vi "Saccade suppression - moving grating by time.vi"() -> ()   [LabVIEW 2013]
uses:
  <vilib>/Platform/TimedLoop/XDataNode/timing_clust.ctl
  <vilib>/Platform/TimedLoop/XDataNode/nitl_modes.ctl
  <vilib>/Platform/TimedLoop/XDataNode/wakeup.ctl
  <vilib>/gmath/statdist.llb/Uniform (Discrete) Random.vi
  Eye tracking dependencies/Global 1.vi
  <vilib>/platform/TimedLoop/XDataNode/XDataNode.xnode
  <vilib>/Platform/TimedLoop/XDataNode/XDNodeRunTimeDep.lvlib
  <vilib>/gmath/NI_Gmath.lvlib
panel:
  out "Eye tracker":bool
  out "Std name":string="70915_animal15-21_exp1"
  out "Blank":bool
  out "Total number of trials":i32=2
  out "Running!":bool=TRUE
  in  "Location":string="E:\\Beh_Data\\"
  out "File name exists!":bool
  out "Current trial #":u16=1
  out "LED":bool
  in  "Abort":bool caption="run-stop"
  in  "File name":string="17"
  in  "Save data":bool
  out "State Missed":bool
  out "VS missed":bool
  out "State busy":bool=TRUE
  out "VS busy":bool=TRUE
  in  "Tab Control":T1(tab)=enum."Network"
  in  "Notes":string
  in  "Start recording @":string
  in  "Inserted probe @":string
  in  "Brain region":string
  in  "Anesthesia @":string
  in  "Anesthesia":string
  in  "Probe configuration":string
  in  "Probe use number":string
  in  "Probe ID":string
  in  "Probe type":string
  in  "Electrode spacing":string
  in  "Electrode area":string
  in  "Penetration angle (to pia)":string
  in  "Penetration coordinates":string
  in  "Penetration distance":string
  in  "Penetration number":string
  in  "Genotype":string
  in  "Transfection":string
  in  "Mass":string
  in  "Sex":string
  in  "Age":string
  in  "Animal ID":string="14-4"
  in  "inter flash interval (ms)":dbl=500.0
  in  "Max jitter (ms)":dbl=500.0
  in  "VS type":string="saccade_grating"
  in  "Background luminance":sgl=40.0
  in  "Pulse amp 0":sgl
  in  "Pulse amp 1":sgl
  in  "Pulse delay (ms)":sgl
  in  "Pulse width (ms)":sgl
  in  "Pulse period":sgl
  in  "Pulse #":sgl
  in  "LED mode":u16(ring) items=["No LED", "Random"]
  in  "Chance (%)":dbl
  in  "# of trials":i32=1
  in  "run-stop":bool=TRUE
  in  "Time (min)":sgl=1.0
  in  "Flash luminance":sgl=100.0
  in  "flash duration (ms)":dbl=16.0
  in  "VS subtype":string="movingByTime"
  in  "Include blanks":bool=TRUE
  in  "# of blank trials":i32=1
  in  "7":bool
  in  "6":bool
  in  "5":bool
  in  "4":bool
  in  "3":bool
  in  "2":bool
  in  "1":bool
  in  "0":bool=TRUE
  in  "Temporal Frequency":sgl=2.0
  in  "Contrast":sgl=1.0
  in  "Spatial Frequency":sgl=0.03
  in  "Give reward":bool
  in  "Manually give shock":bool
  in  "Water duration (ms)":u32=30
  in  "Shock duration (ms)":u32=10
  in  "Water refractory period (ms)":u32=500
  in  "Shock refractory period (ms)":u32=1000
  in  "Trial timeout (ms)":u32=3000
  in  "Track eye":bool=TRUE
  in  "Allow shock":bool
  in  "Allow timeout":bool
  in  "Manually give water":bool
  in  "Reward period (ms)":u32
  in  "Reward start delay (ms)":u32
  in  "Lick threshold (V)":fxp<+,32,16>=1.600006103515625
  in  "VS threshold (V)":fxp<+,32,16>=0.5
  out "Originating IP":string="192.168.137.2"
  out "Incoming data":string="TrlDone 1.000 "
  in  "Update cycle (ms)":dbl=50.0
  in  "Local IP_This computer":string="192.168.137.10"
  in  "Remote IP_Broadcast":string="192.168.137.255"
  in  "Remote IP_State machine":string="192.168.137.2"
  in  "Remote IP_Visual stimulation":string="192.168.137.3"
  in  "Local port":u16=9090
  in  "Remote port":u16=9091
  out "Error 2":string
  # "Saccade suppression project"
  # "Current trial"
  # "of"
  # "System Status"
  # "VS"
  # "State machine"
  # "Busy"
  # "Missed trial"
  # "Max 20 characters"
  # "(w/o LED)"
  # "Time per trial (min)"
  # "MAX 199.9988"
  # "(% of blank trials that have LED)"
  # "Errors for debugging"
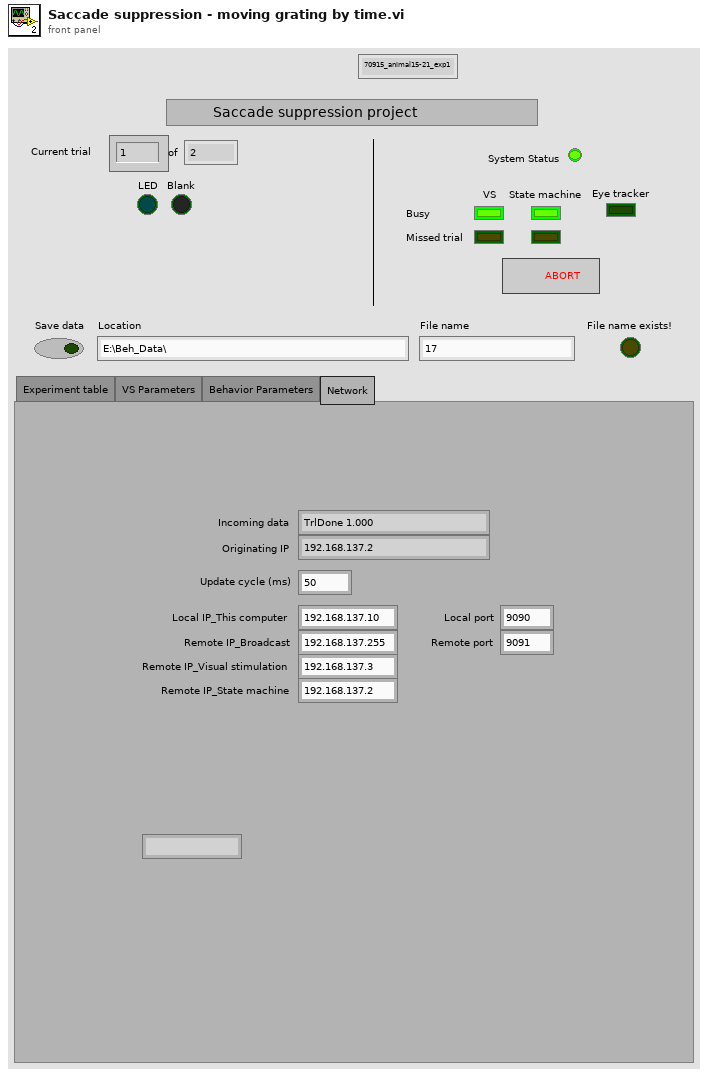
[diagram p1: front panel]
types:
  T1 = enum32{"Experiment table", "VS Parameters", "Behavior Parameters", "Network"}
  T2 = typedef "XDNodeRunTimeDep.lvlib/timing_clust.ctl" = cluster{"Expected End [f-1]":u64, "Actual End [f-1]":u64, "Finished Late? [f-1]":bool, "Expected End [i-1]":u64, "Actual End [i-1]":u64, "Finished Late? [i-1]":bool, "Expected Start [i]":u64, "Actual Start [i]":u64, "Expected Start [f]":u64, "Actual Start [f]":u64, "Source Name":string, "Structure Name":string, "Period":i64, "Deadline":i64, "Offset":i64, "Start":i64, "Priority":i32, "Timeout":i32, "Mode":T3, "Wakeup Reason":T4, "Error":errorcluster, "Source Type":string, "Secondary Source Type":string, "Global End Time":u64, "Global Start Time":u64, "Frame Duration":u64, "Iteration Duration":u64, "Assigned CPU":i32, "I/O Scan Engine Mode":u32}
  T3 = typedef "XDNodeRunTimeDep.lvlib/nitl_modes.ctl" = enum32{"No Change", "Process missed periods, maintain original phase", "Discard missed periods, maintain original phase", "Process missed periods, ignore original phase", "Discard missed periods, ignore original phase"}
  T4 = typedef "XDNodeRunTimeDep.lvlib/wakeup.ctl" = enum32{"Normal", "Aborted", "Asynchronous wakeup", "Timing source error", "Timed loop error", "Timeout"}
  T5 = enum16{"big-endian, network order", "native, host order", "little-endian"}
  T6 = enum16{"open", "replace", "create", "open or create", "replace or create", "replace or create with confirmation"}
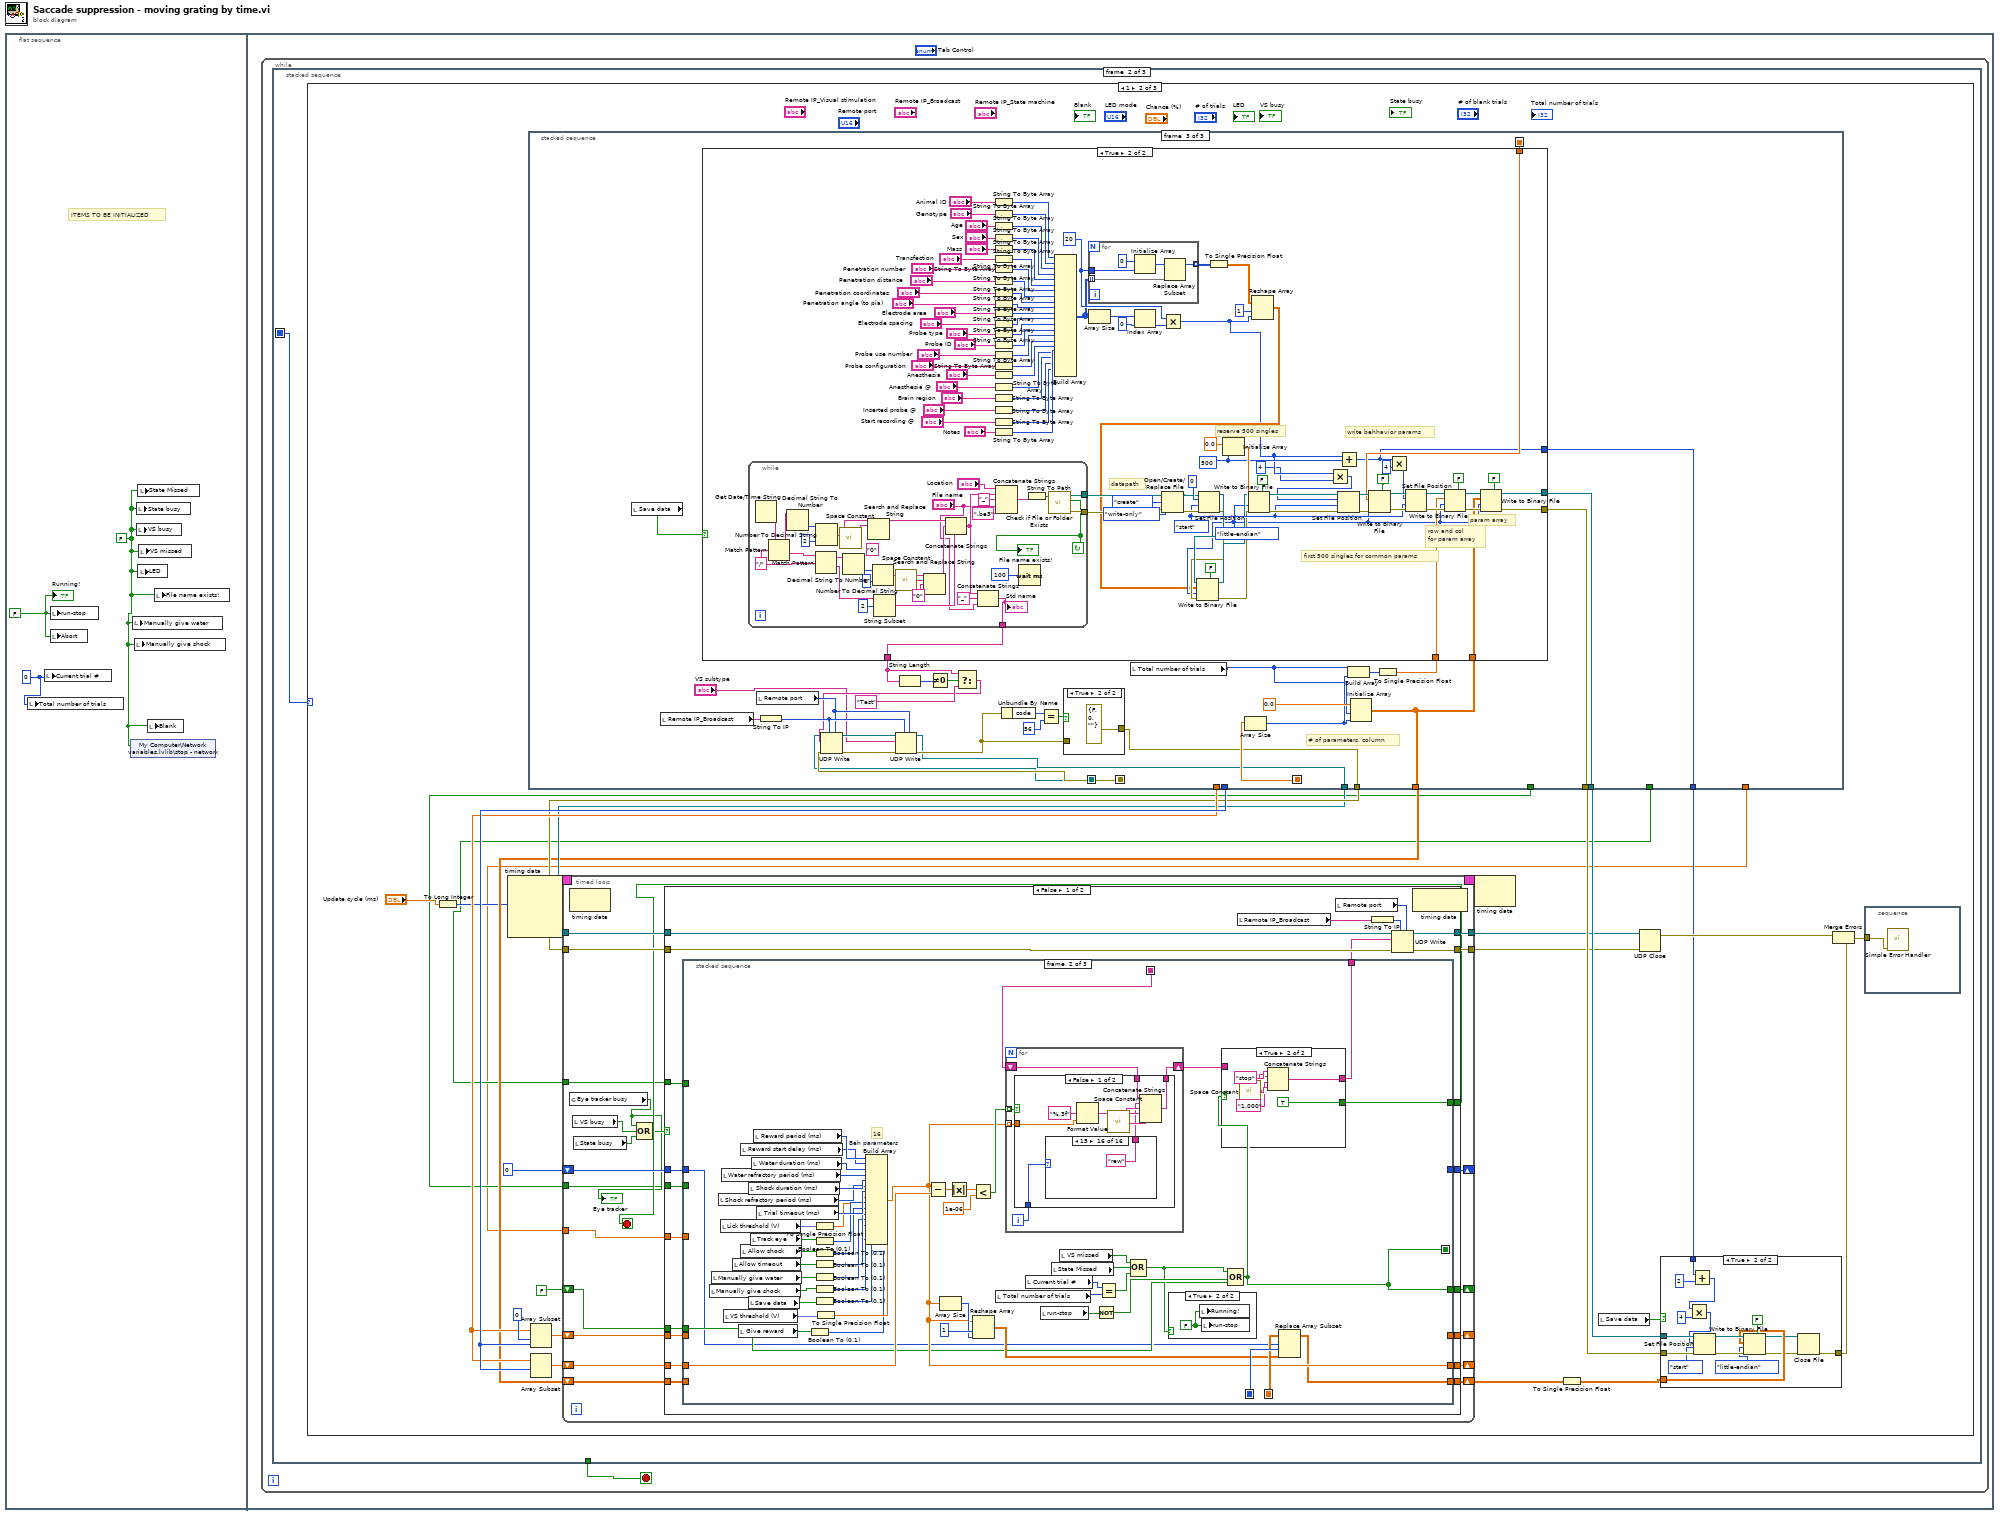
[diagram p0: block diagram]
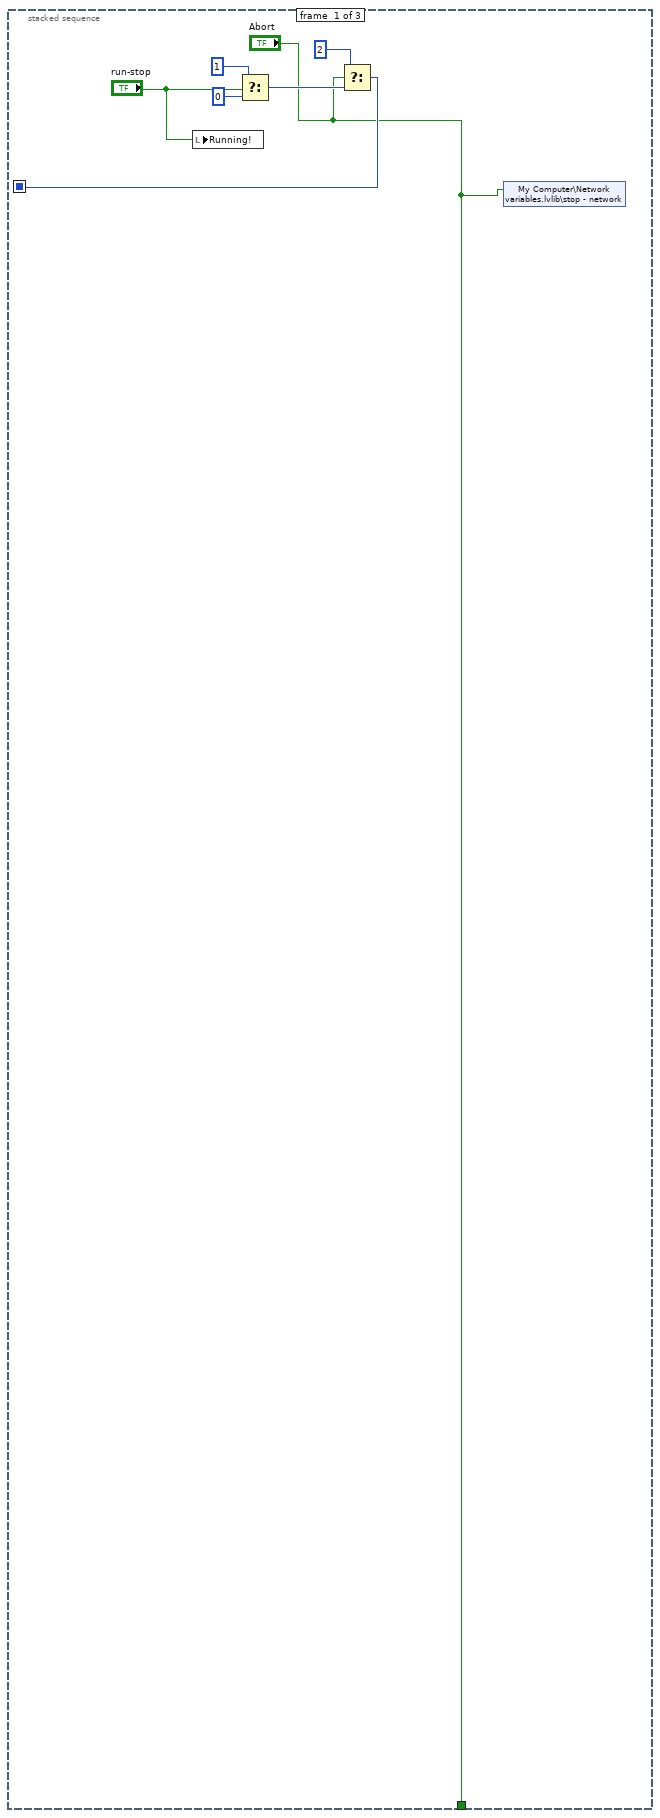
[diagram p2: hidden frame]
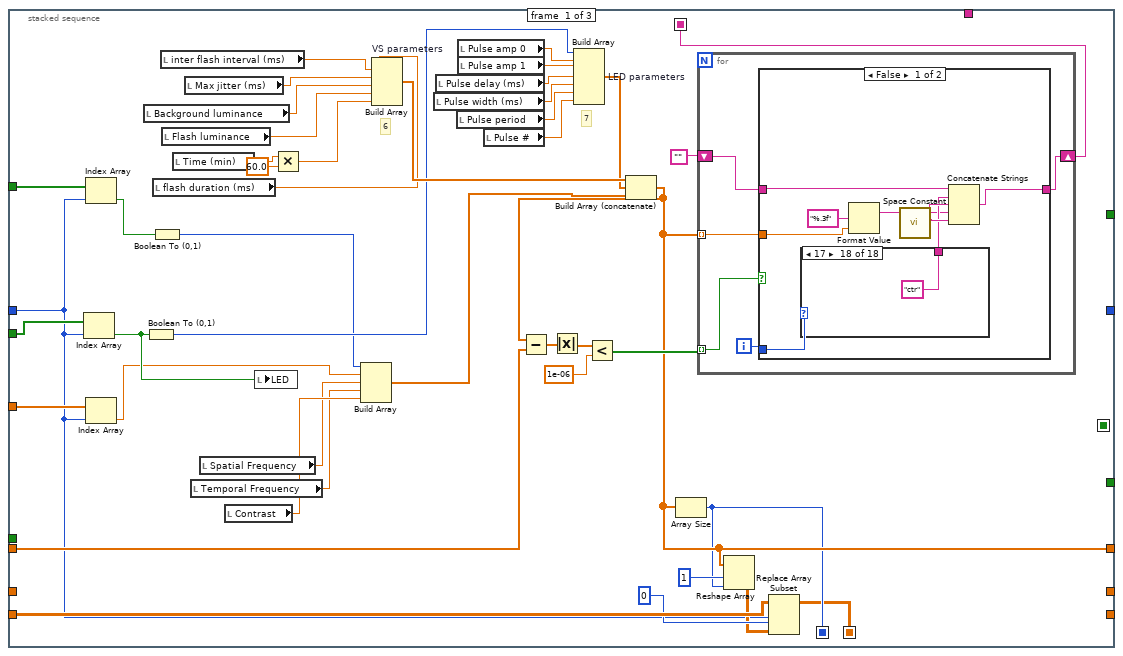
[diagram p4: hidden frame]
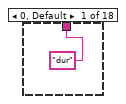
[diagram p5: hidden frame]
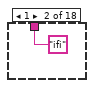
[diagram p6: hidden frame]
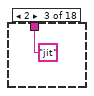
[diagram p7: hidden frame]
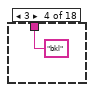
[diagram p8: hidden frame]
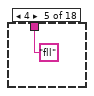
[diagram p9: hidden frame]
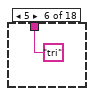
[diagram p10: hidden frame]
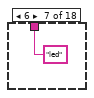
[diagram p11: hidden frame]
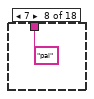
[diagram p12: hidden frame]
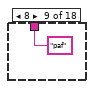
[diagram p13: hidden frame]
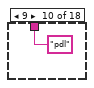
[diagram p14: hidden frame]
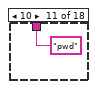
[diagram p15: hidden frame]
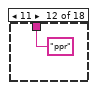
[diagram p16: hidden frame]
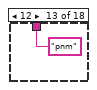
[diagram p17: hidden frame]
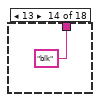
[diagram p18: hidden frame]
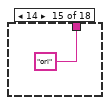
[diagram p19: hidden frame]
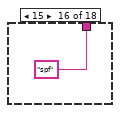
[diagram p20: hidden frame]
diagram:
  n1 = flat-sequence {
    frame #0 {
      w2 = u16 0
      w1 = FALSE ("L dist ind")
      w3 = FALSE
      # "ITEMS TO BE INITIALIZED"
      n2 = local write "Total number of trials"(w2) -> ()
      n3 = local write "Current trial #"(w2) -> ()
      n4 = local write "run-stop"(w3) -> ()
      n5 = local write "Abort"(w3) -> ()
      n6 = shared-variable "My Computer\\Network variables.lvlib\\stop - network"(w1) -> ()  [unwired: 1 in, 1 out]
      n7 = local write "Manually give water"(w1) -> ()
      n8 = local write "Manually give shock"(w1) -> ()
      n9 = local write "State busy"(w1) -> ()
      n10 = local write "VS busy"(w1) -> ()
      n11 = local write "State Missed"(w1) -> ()
      n12 = local write "LED"(w1) -> ()
      n13 = local write "VS missed"(w1) -> ()
      n14 = local write "Blank"(w1) -> ()
      n15 = local write "File name exists!"(w1) -> ()
      "Running!" <- w3
    }
    frame #1 {
      n16 = while {
        stop <- w4 stop-if-true
        n17 = stacked-sequence {
          seq-local: [w7 _ _] -> [_ w12 _]
          tunnel: ["Abort" _ _] -> w4
          frame #0 {
            n18 = local write "Running!"("run-stop") -> ()
            n19 = Select(t=u8 1, s="run-stop", f=u8 0) -> (s? t:f=w8:u8)
            n20 = Select(t=u8 2, s="Abort", f=w8) -> (s? t:f=w7:u8)
            n21 = shared-variable "My Computer\\Network variables.lvlib\\stop - network"("Abort") -> ()  [unwired: 1 in, 1 out]
          }
          frame #1 {
            n22 = case shown="1" w12 {
              frame 0, Default {
              }
              frame 1 {
                n23 = To Long Integer(number="Update cycle (ms)") -> (32bit integer=w23:i32)
                n24 = node-c288(w23) -> (w40:T2)  [unwired: 3 in]
                n25 = stacked-sequence {
                  seq-local: [w464 _ _] -> [_ _ w676]
                  seq-local: [_ w618 _] -> [_ _ w667]
                  seq-local: [w473 _ _] -> [_ _ w665]
                  seq-local: [w472 _ _] -> [_ _ w651]
                  tunnel: [w464 _ _] -> w35
                  tunnel: [w461 _ _] -> w36
                  tunnel: [_ _ w649] -> w32
                  tunnel: [_ _ w648] -> w31
                  tunnel: [_ _ w670] -> w30
                  tunnel: [_ _ w669] -> w26
                  tunnel: [_ _ w668] -> w25
                  tunnel: [_ _ w646] -> w16
                  tunnel: [w457 _ _] -> w15
                  tunnel: [w456 _ _] -> w14
                  tunnel: [w448 _ _] -> w13
                  frame #0 {
                    # "5"
                    # "Orientation"
                    n26 = Boolean To (0,1)(Boolean="Give reward") -> (0, 1=w474:i16)
                    n27 = Boolean To (0,1)(Boolean="Track eye") -> (0, 1=w514:i16)
                    n28 = To Single Precision Float(number="Lick threshold (V)") -> (single precision float=w479:sgl)
                    n29 = Boolean To (0,1)(Boolean="Allow shock") -> (0, 1=w512:i16)
                    n30 = Boolean To (0,1)(Boolean="Allow timeout") -> (0, 1=w510:i16)
                    n31 = Boolean To (0,1)(Boolean="Manually give water") -> (0, 1=w508:i16)
                    n32 = Boolean To (0,1)(Boolean="Save data") -> (0, 1=w505:i16)
                    n33 = To Single Precision Float(number="VS threshold (V)") -> (single precision float=w476:sgl)
                    n34 = Boolean To (0,1)(Boolean="Manually give shock") -> (0, 1=w507:i16)
                    n35 = Build Array "Beh parameters 16"("Reward period (ms)", "Reward start delay (ms)", "Water duration (ms)", "Water refractory period (ms)", "Shock duration (ms)", "Shock refractory period (ms)", "Trial timeout (ms)", w479, w514, w512, w510, w508, w507, w505, w476, w474) -> (w463:sgl[])
                    n36 = local read "Remote IP_Broadcast"() -> (w492:string)
                    n37 = String To IP(1:"Local IP_This computer") -> (0:w496:u32)
                    n38 = UDP Open(7:w496, 11:"Local port") -> (port=w493:refnum<k16>, 0:w497:errorcluster)  [unwired: 3 in, 1 out]
                    n39 = local read "Remote port"() -> (w487:u16)
                    n40 = Multiply(x="Time (min)", y=sgl 60.0) -> (x*y=w454:sgl)
                    n41 = String To IP(1:w492) -> (0:w488:u32)
                    n42 = Build Array "VS parameters 6"("flash duration (ms)", "inter flash interval (ms)", "Max jitter (ms)", "Background luminance", "Flash luminance", w454) -> (w483:dbl[])
                    n43 = Array Size(array=w483) -> (size(s)=w481:i32)
                    n44 = call <vilib>:"Space Constant.vi"() -> ("String"=w490:string)
                    n45 = stacked-sequence {
                      tunnel: [w525 _] -> w457
                      tunnel: [w524 _] -> w456
                      tunnel: [_ w578] -> w448
                      frame #0 {
                        n46 = case shown="True" "Include blanks" {
                          tunnel: [w529 w532] -> w525
                          tunnel: [w527 w534] -> _
                          tunnel: [w526 w533] -> w524
                          frame False {
                            n47 = local read "# of trials"() -> (w527:i32)
                            n48 = Initialize Array(FALSE, w527) -> (w526:bool[])
                            n49 = Initialize Array(FALSE, w527) -> (w529:bool[])
                            n50 = local write "Total number of trials"(w527) -> ()
                          }
                          frame True {
                            n51 = local read "LED mode"() -> (w535:u16)
                            n52 = local read "# of blank trials"() -> (w531:i32)
                            n53 = local read "# of trials"() -> (w536:i32)
                            n54 = Add(x=w536, y=w531) -> (x+y=w534:i32)
                            n55 = local write "Total number of trials"(w534) -> ()
                            n56 = Initialize Array(FALSE, w536) -> (w537:bool[])
                            n57 = for {
                              N: w531 -> [_]
                              shift-right: [w571] -> w532
                              shift-left: w537 -> [w572]
                              n58 = Array Size(array=w572) -> (size(s)=w576:i32)
                              n59 = call-poly <vilib>:"Discrete Random.vi"("n"=w576, "samples"=1) -> ("uniform (discrete) random data"=w575:i32[])  [unwired: 8 in, 1 out]
                              n60 = Index Array(array=w575, index=0) -> (element=w573:i32)
                              n61 = Decrement(x=w573) -> (x-1=w570:i32)
                              n62 = Insert Into Array(array=w572, index=w570, new element=TRUE) -> (w571:bool[])
                            }
                            n63 = case shown="1" w535 {
                              tunnel: w534 -> [w541 w543]
                              tunnel: [w540 w544] -> w533
                              tunnel: w532 -> [_ w549]
                              tunnel: w531 -> [_ _]
                              frame 0, Default {
                                n64 = Initialize Array(FALSE, w541) -> (w540:bool[])
                              }
                              frame 1 {
                                n65 = local read "Chance (%)"() -> (w547:dbl)
                                n66 = Decrement(x=w543) -> (x-1=w542:i32)
                                n67 = Divide(x=w547, y=100.0) -> (x/y=w545:dbl)
                                n68 = while {
                                tunnel: w549 -> [w557]
                                shift-right: [w555] -> w544
                                shift-left: bool[] [] -> [w554]
                                tunnel: w545 -> [w553]
                                tunnel: w542 -> [w551]
                                i -> [w552]
                                stop <- w550 stop-if-true
                                n69 = Index Array(array=w557, index=w552) -> (element=w556:bool)
                                n70 = Equal?(x=w552, y=w551) -> (x = y?=w550:bool)
                                n71 = case shown="True" w556 {
                                tunnel: [w559 w568] -> w555
                                tunnel: w554 -> [w558 w567]
                                tunnel: w553 -> [_ w562]
                                frame False {
                                n72 = Build Array (concatenate)(w558, FALSE) -> (w559:bool[])
                                }
                                frame True {
                                n73 = Random Number (0-1)() -> (number: 0 to 1=w561:dbl)
                                n74 = Less?(x=w561, y=w562) -> (x < y?=w563:bool)
                                n75 = Select(t=TRUE, s=w563, f=FALSE) -> (s? t:f=w566:bool)
                                n76 = Build Array (concatenate)(w567, w566) -> (w568:bool[])
                                }
                                }
                                }
                              }
                            }
                          }
                        }
                      }
                      frame #1 {
                        n77 = local read "Total number of trials"() -> (w580:i32)
                        n78 = for {
                          N: w580 -> [_]
                          shift-right: [w581] -> w578
                          shift-left: sgl[] [] ("array type (2D Dbl)") -> [w582]
                          n79 = Boolean To (0,1)(Boolean="6") -> (0, 1=w590:i16)
                          n80 = Boolean To (0,1)(Boolean="7") -> (0, 1=w589:i16)
                          n81 = Boolean To (0,1)(Boolean="5") -> (0, 1=w591:i16)
                          n82 = Boolean To (0,1)(Boolean="4") -> (0, 1=w592:i16)
                          n83 = Boolean To (0,1)(Boolean="0") -> (0, 1=w596:i16)
                          n84 = Boolean To (0,1)(Boolean="1") -> (0, 1=w595:i16)
                          n85 = Boolean To (0,1)(Boolean="3") -> (0, 1=w593:i16)
                          n86 = Boolean To (0,1)(Boolean="2") -> (0, 1=w594:i16)
                          n87 = Compound Arithmetic op=ADD(w596, w595, w594, w593, w592, w591, w590, w589) -> (w588:i16)
                          n88 = Build Array(w596, w595, w594, w593, w592, w591, w590, w589) -> (w587:i16[])
                          n89 = call-poly <vilib>:"Discrete Random.vi"("n"=w588, "samples"=1) -> ("uniform (discrete) random data"=w607:i32[])  [unwired: 8 in, 1 out]
                          n90 = Index Array(array=w607, index=0) -> (element=w605:i32)
                          n91 = Decrement(x=w605) -> (x-1=w586:i32)
                          n92 = while {
                            tunnel: w587 -> [w616]
                            tunnel: [w614] -> w584
                            tunnel: w586 -> [w612]
                            shift-right: [w609] -> _
                            shift-left: 0 -> [w610]
                            i -> [w613]
                            stop <- w611 stop-if-true
                            n93 = Search 1D Array(1D array=w616, element=i16 1, start index (0)=w610) -> (index of element=w614:i32)
                            n94 = Equal?(x=w613, y=w612) -> (x = y?=w611:bool)
                            n95 = Increment(x=w614) -> (x+1=w609:i32)
                          }
                          n96 = To Single Precision Float(number=w584) -> (single precision float=w583:sgl)
                          n97 = Build Array (concatenate)(w582, w583) -> (w581:sgl[])
                        }
                      }
                    }
                    n98 = Index Array(array=w448, index=0) -> (element=w450:sgl)
                    n99 = Index Array(array=w456, index=0) -> (element=w459:bool)
                    n100 = Index Array(array=w457, index=0) -> (element=w465:bool)
                    n101 = Boolean To (0,1)(Boolean=w459) -> (0, 1=w458:i16)
                    n102 = Build Array "LED parameters 7"(w458, "Pulse amp 0", "Pulse amp 1", "Pulse delay (ms)", "Pulse width (ms)", "Pulse period", "Pulse #") -> (w482:sgl[])
                    n103 = Array Size(array=w482) -> (size(s)=w480:i32)
                    n104 = Add(x=w481, y=w480) -> (x+y=w462:i32)
                    n105 = Increment(x=w462) -> (x+1=w461:i32)
                    n106 = Boolean To (0,1)(Boolean=w465) -> (0, 1=w451:i16)
                    n107 = Build Array(w451, w450, "Spatial Frequency", "Temporal Frequency", "Contrast") -> (w452:sgl[])
                    n108 = Build Array (concatenate)(w483, w482, w452, w463) -> (w464:dbl[])
                    n109 = Array To Spreadsheet String(delimiter (Tab)=w490, array=w464, 3:"%.3f" ("format string")) -> (spreadsheet string=w489:string)
                    n110 = UDP Write(address=w488, port or service name=w487, connection ID=w493, data in=w489, 8:w497) -> (error out=w486:errorcluster, 3:w485:refnum<k16>)  [unwired: 1 in]
                    n111 = UDP Write(address=w488, port or service name=w487, connection ID=w485, data in="VS type", 8:w486) -> (error out=w473:errorcluster, 3:w472:refnum<k16>)  [unwired: 1 in]
                  }
                  frame #1 {
                    w625 = "&" ("string")
                    # "state definition"
                    n112 = local read "inter flash interval (ms)"() -> (w640:dbl)
                    n113 = local read "Total number of trials"() -> (w617:i32)
                    n114 = local read "Max jitter (ms)"() -> (w639:dbl)
                    n115 = local read "VS subtype"() -> (w644:string)
                    n116 = local read "Chance (%)"() -> (w638:dbl)
                    n117 = local read "LED mode"() -> (w641:u16)
                    n118 = local read "VS type"() -> (w645:string)
                    n119 = String To Byte Array(string=w645) -> (unsigned byte array=w643:u8[])
                    n120 = String To Byte Array(string=w644) -> (unsigned byte array=w642:u8[])
                    n121 = Concatenate Strings("idle", w625, "vs before", w625, "vs", w625, "vs after", w625, "cycle end", w625, "reward", w625, "reward refractory", w625, "punish", w625, "punish refractory", w625, "exit", w625, "timeout", w625) -> (w626:string)
                    n122 = Build Array (concatenate)(w643, w642, w641, w617, w640, w639, w638) -> (w622:dbl[])
                    n123 = String To Byte Array(string=w626) -> (unsigned byte array=w620:u8[])
                    n124 = Initialize Array(sgl 0.0 ("element"), 37 ("dimension size")) -> (w621:sgl[])
                    n125 = Build Array (concatenate)(w622, w621, w620) -> (w619:dbl[])
                    n126 = To Single Precision Float(number=w619) -> (single precision float=w618:sgl[])
                  }
                  frame #2 {
                    # "# of parameters, column"
                    n127 = local read "Save data"() -> (w673:bool)
                    n128 = local read "Remote IP_Broadcast"() -> (w659:string)
                    n129 = local read "Remote port"() -> (w657:u16)
                    n130 = String To IP(1:w659) -> (0:w658:u32)
                    n131 = local read "Total number of trials"() -> (w666:i32)
                    n132 = Array Size(array=w676) -> (size(s)=w674:i32)
                    n133 = Build Array(w666, w674) -> (w672:i32[])
                    n134 = Initialize Array(sgl 0.0, w666, w674) -> (w670:sgl[][])
                    n135 = To Single Precision Float(number=w672) -> (single precision float=w671:sgl[])
                    n136 = case shown="True" w673 {
                      tunnel: w671 -> [_ w749]
                      tunnel: w670 -> [_ w748]
                      tunnel: [_ w747] -> w669
                      tunnel: [_ w746] -> w668
                      tunnel: w667 -> [_ w745]
                      tunnel: ["" w681] -> w653
                      tunnel: [_ w680] -> w646
                      frame False {
                      }
                      frame True {
                        w716 = 20 ("dimension size")
                        w686 = 500 ("dimension size")
                        w688 = T5."little-endian" ("byte order (0:big-endian, network order)")
                        w758 = enum16{"start", "end", "current"}."start" ("from (0:start)")
                        # "param array"
                        # "row and col\nfor param array"
                        # "first 500 singles for common params"
                        # "reserve 500 singles"
                        # "write behhavior params"
                        # "datapath"
                        n137 = while {
                          tunnel: [w789] -> w751
                          tunnel: [w788] -> w750
                          tunnel: [w781] -> w681
                          stop <- w786 continue-if-true
                          (unwired) "0" ("replace string (\"\")")
                          w810 = "/"
                          n138 = Get Date/Time String() -> (date string=w812:string)  [unwired: 3 in, 1 out]
                          n139 = Match Pattern(string=w812, regular expression=w810) -> (before substring=w809:string, after substring=w811:string)  [unwired: 1 in, 2 out]
                          n140 = Decimal String To Number(string=w809) -> (number=w804:i32)  [unwired: 2 in, 1 out]
                          n141 = Match Pattern(string=w811, regular expression=w810) -> (before substring=w808:string, after substring=w798:string)  [unwired: 1 in, 2 out]
                          n142 = Number To Decimal String(number=w804, width (-)=i16 2) -> (decimal integer string=w806:string)
                          n143 = call <vilib>:"Space Constant.vi"() -> ("String"=w805:string)
                          n144 = Decimal String To Number(string=w808) -> (number=w801:i32)  [unwired: 2 in, 1 out]
                          n145 = Search and Replace String(input string=w806, search string=w805) -> (result string=w796:string)  [unwired: 6 in, 3 out]
                          n146 = Number To Decimal String(number=w801, width (-)=i16 2) -> (decimal integer string=w803:string)
                          n147 = String Subset(string=w798, offset (0)=2) -> (substring=w794:string)  [unwired: 1 in]
                          n148 = call <vilib>:"Space Constant.vi"() -> ("String"=w802:string)
                          n149 = Search and Replace String(input string=w803, search string=w802, replace string="0" ("replace string (\"\")")) -> (result string=w795:string)  [unwired: 5 in, 3 out]
                          n150 = Concatenate Strings(w796, w795, w794) -> (w784:string)
                          n151 = Concatenate Strings(w784, "_" ("string"), "File name") -> (w781:string)
                          "Std name" <- w781
                          n152 = Concatenate Strings("Location", w784, "_" ("string"), "File name", ".be3" ("string")) -> (w791:string)
                          n153 = Wait (ms)(milliseconds to wait=u32 100) -> ()  [unwired: 1 out]
                          n154 = String To Path(string=w791) -> (path=w790:path)
                          n155 = call <vilib>:"Check if File or Folder Exists.vi"("path"=w790) -> ("error out"=w788:errorcluster, "file or folder exists?"=w786:bool, "dup path"=w789:path)  [unwired: 8 in]
                          "File name exists!" <- w786
                        }
                        n156 = String To Byte Array(string="Animal ID") -> (unsigned byte array=w708:u8[])
                        n157 = String To Byte Array(string="Genotype") -> (unsigned byte array=w699:u8[])
                        n158 = String To Byte Array(string="Age") -> (unsigned byte array=w700:u8[])
                        n159 = String To Byte Array(string="Sex") -> (unsigned byte array=w701:u8[])
                        n160 = String To Byte Array(string="Mass") -> (unsigned byte array=w702:u8[])
                        n161 = String To Byte Array(string="Transfection") -> (unsigned byte array=w703:u8[])
                        n162 = String To Byte Array(string="Penetration number") -> (unsigned byte array=w705:u8[])
                        n163 = String To Byte Array(string="Penetration distance") -> (unsigned byte array=w707:u8[])
                        n164 = String To Byte Array(string="Penetration coordinates") -> (unsigned byte array=w731:u8[])
                        n165 = String To Byte Array(string="Penetration angle (to pia)") -> (unsigned byte array=w732:u8[])
                        n166 = String To Byte Array(string="Electrode area") -> (unsigned byte array=w733:u8[])
                        n167 = String To Byte Array(string="Electrode spacing") -> (unsigned byte array=w734:u8[])
                        n168 = String To Byte Array(string="Probe type") -> (unsigned byte array=w735:u8[])
                        n169 = String To Byte Array(string="Probe ID") -> (unsigned byte array=w736:u8[])
                        n170 = String To Byte Array(string="Probe use number") -> (unsigned byte array=w737:u8[])
                        n171 = String To Byte Array(string="Probe configuration") -> (unsigned byte array=w738:u8[])
                        n172 = String To Byte Array(string="Anesthesia") -> (unsigned byte array=w739:u8[])
                        n173 = String To Byte Array(string="Anesthesia @") -> (unsigned byte array=w740:u8[])
                        n174 = String To Byte Array(string="Brain region") -> (unsigned byte array=w741:u8[])
                        n175 = String To Byte Array(string="Inserted probe @") -> (unsigned byte array=w742:u8[])
                        n176 = String To Byte Array(string="Start recording @") -> (unsigned byte array=w743:u8[])
                        n177 = String To Byte Array(string="Notes") -> (unsigned byte array=w744:u8[])
                        n178 = Build Array(w708, w699, w700, w701, w702, w703, w705, w707, w731, w732, w733, w734, w735, w736, w737, w738, w739, w740, w741, w742, w743, w744) -> (w711:u8[][])
                        n179 = for {
                          tunnel: w711 -> [w778] mode=indexing
                          tunnel: [w777] -> w709 mode=indexing
                          tunnel: w716 -> [w776]
                          n180 = Initialize Array(u8 0 ("element"), w776) -> (w780:u8[])
                          n181 = Replace Array Subset(array=w780, new element=w778) -> (w777:u8[])  [unwired: 1 in]
                        }
                        n182 = Array Size(array=w711) -> (size(s)=w713:i32[])
                        n183 = Index Array(array=w713, index=0) -> (element=w715:i32)
                        n184 = Open/Create/Replace File(file path (use dialog)=w751, error in=w750, operation (0:open)=T6."create", access (0:read/write)=enum16{"read/write", "read-only", "write-only"}."write-only") -> (refnum out=w772:refnum<file>, error out=w771:errorcluster)  [unwired: 2 in, 1 out]
                        n185 = Multiply(x=w716, y=w715) -> (x*y=w684:i32)
                        n186 = Set File Position(offset (in bytes) (0)=i64 0, refnum=w772, from (0:start)=w758, error in=w771) -> (refnum out=w692:refnum<file>, error out=w690:errorcluster)
                        n187 = To Single Precision Float(number=w709) -> (single precision float=w710:sgl[][])
                        n188 = Initialize Array(sgl 0.0 ("element"), w686) -> (w768:sgl[])
                        n189 = Reshape Array(w710, 1 ("dimension size"), w684) -> (w687:sgl[][])
                        n190 = Write to Binary File(file (use dialog)=w692, data=w687, error in=w690, 5:FALSE ("prepend array or string size? (T)"), 9:w688) -> (refnum out=w691:refnum<file>, error out=w689:errorcluster)  [unwired: 1 in, 1 out]
                        n191 = Write to Binary File(file (use dialog)=w691, data=w768, error in=w689, 5:FALSE ("prepend array or string size? (T)"), 9:w688) -> (refnum out=w766:refnum<file>, error out=w765:errorcluster)  [unwired: 1 in, 1 out]
                        n192 = Multiply(x=w684, y=4) -> (x*y=w685:i32)
                        n193 = Set File Position(offset (in bytes) (0)=w685, refnum=w766, from (0:start)=w758, error in=w765) -> (refnum out=w764:refnum<file>, error out=w763:errorcluster)
                        n194 = Add(x=w684, y=w686) -> (x+y=w680:i32)
                        n195 = Write to Binary File(file (use dialog)=w764, data=w745, error in=w763, 5:FALSE ("prepend array or string size? (T)"), 9:w688) -> (refnum out=w762:refnum<file>, error out=w761:errorcluster)  [unwired: 1 in, 1 out]
                        n196 = Multiply(x=w680, y=4) -> (x*y=w760:i32)
                        n197 = Set File Position(offset (in bytes) (0)=w760, refnum=w762, from (0:start)=w758, error in=w761) -> (refnum out=w756:refnum<file>, error out=w755:errorcluster)
                        n198 = Write to Binary File(file (use dialog)=w756, data=w749, error in=w755, 5:FALSE ("prepend array or string size? (T)"), 9:w688) -> (refnum out=w754:refnum<file>, error out=w753:errorcluster)  [unwired: 1 in, 1 out]
                        n199 = Write to Binary File(file (use dialog)=w754, data=w748, error in=w753, 5:FALSE ("prepend array or string size? (T)"), 9:w688) -> (refnum out=w746:refnum<file>, error out=w747:errorcluster)  [unwired: 1 in, 1 out]
                      }
                    }
                    n200 = String Length(string=w653) -> (length=w656:i32)
                    n201 = Not Equal To 0?(x=w656) -> (x != 0?=w655:bool)
                    n202 = Select(t=w653, s=w655, f="Test") -> (s? t:f=w652:string)
                    n203 = UDP Write(address=w658, port or service name=w657, connection ID=w651, data in=w652, 8:w665) -> (error out=w664:errorcluster, 3:w650:refnum<k16>)  [unwired: 1 in]
                    n204 = UDP Write(address=w658, port or service name=w657, connection ID=w650, data in="VS subtype", 8:w664) -> (error out=w660:errorcluster, 3:w648:refnum<k16>)  [unwired: 1 in]
                    n205 = Unbundle By Name(w660) -> ("code"=w663:i32)
                    n206 = Equal?(x=w663, y=56) -> (x = y?=w661:bool)
                    n207 = case shown="True" w661 {
                      tunnel: w660 -> [w677 _]
                      tunnel: [w677 errorcluster {"status"=FALSE, "code"=0, "source"=""} ("error out")] -> w649
                      frame False {
                      }
                      frame True {
                      }
                    }
                  }
                }
                n208 = Array Subset(array=w35, index=0, length=w36) -> (w38:dbl[])
                n209 = Array Subset(array=w35, index=w36) -> (w34:dbl[])  [unwired: 1 in]
                n210 = timed-loop {
                  shift-right: [w61] -> _
                  shift-left: u16 0 -> [w60]
                  tunnel: w32 -> [w59]
                  tunnel: w31 -> [w58]
                  tunnel: [w57] -> w17
                  tunnel: [w56] -> w18
                  shift-right: [w55] -> _
                  shift-left: w38 -> [w63]
                  shift-right: [w54] -> _
                  shift-left: w34 -> [w62]
                  shift-right: [w52] -> w29
                  shift-left: w30 -> [w53]
                  shift-right: [w51] -> _
                  shift-left: FALSE -> [w50]
                  timing: w40 -> [_]
                  timing-out: [_] -> w39
                  tunnel: w15 -> [w44]
                  tunnel: w14 -> [w43]
                  tunnel: w13 -> [w42]
                  stop <- w49 stop-if-true
                  n211 = node-c288() -> ()  [unwired: 1 in, 1 out]
                  n212 = global read "Global 1.vi" "Eye tracker busy"() -> (w45:bool)
                  "Eye tracker" <- w45
                  n213 = local read "VS busy"() -> (w47:bool)
                  n214 = local read "State busy"() -> (w46:bool)
                  n215 = Compound Arithmetic op=OR(w45, w47, w46) -> (w48:bool)
                  n216 = case shown="False" w48 {
                    tunnel: w63 -> [w87 w277]
                    tunnel: w62 -> [w86 w275]
                    tunnel: [w85 w266] -> w61
                    tunnel: w60 -> [w84 w267]
                    tunnel: w59 -> [w80 w273]
                    tunnel: w58 -> [w79 w271]
                    tunnel: [w78 w272] -> w57
                    tunnel: [w77 w270] -> w56
                    tunnel: [w76 w277] -> w55
                    tunnel: [w75 w268] -> w54
                    tunnel: w53 -> [w74 w276]
                    tunnel: [w73 w276] -> w52
                    tunnel: [w72 w269] -> w51
                    tunnel: w50 -> [w71 w274]
                    tunnel: [w69 FALSE] -> w49
                    tunnel: w44 -> [w68 _]
                    tunnel: w43 -> [w67 _]
                    tunnel: w42 -> [w66 _]
                    frame False {
                      n217 = stacked-sequence {
                        seq-local: [w117 _ _] -> [_ w188 _]
                        seq-local: [w110 _ _] -> [_ w182 _]
                        seq-local: [w109 _ _] -> [_ w181 _]
                        seq-local: [_ w171 _] -> [_ _ w258]
                        tunnel: w84 -> [w94 w169 w260]
                        tunnel: w87 -> [w122 _ _]
                        tunnel: w86 -> [_ w195 _]
                        tunnel: [_ _ w259] -> w85
                        tunnel: [w114 _ _] -> w76
                        tunnel: [_ w178 _] -> w75
                        tunnel: w74 -> [w113 _ _]
                        tunnel: [_ w176 _] -> w73
                        tunnel: [_ w171 _] -> w72
                        tunnel: w71 -> [_ w172 _]
                        tunnel: [_ w170 _] -> w70
                        tunnel: [_ w163 _] -> w69
                        tunnel: w68 -> [w103 _ _]
                        tunnel: w67 -> [w101 _ _]
                        tunnel: w66 -> [w95 _ _]
                        frame #0 {
                          # "6"
                          # "7"
                          n218 = Index Array(array=w101, index=w94) -> (element=w99:bool)
                          n219 = Index Array(array=w103, index=w94) -> (element=w102:bool)
                          n220 = Index Array(array=w95, index=w94) -> (element=w90:sgl)
                          n221 = local read "Background luminance"() -> (w106:sgl)
                          n222 = Boolean To (0,1)(Boolean=w99) -> (0, 1=w100:i16)
                          n223 = Boolean To (0,1)(Boolean=w102) -> (0, 1=w89:i16)
                          n224 = local read "flash duration (ms)"() -> (w104:dbl)
                          n225 = local read "inter flash interval (ms)"() -> (w108:dbl)
                          n226 = local read "Flash luminance"() -> (w105:sgl)
                          n227 = local read "Time (min)"() -> (w97:sgl)
                          n228 = local read "Max jitter (ms)"() -> (w107:dbl)
                          n229 = local read "Temporal Frequency"() -> (w92:sgl)
                          n230 = local read "Spatial Frequency"() -> (w91:sgl)
                          n231 = local read "Contrast"() -> (w93:sgl)
                          n232 = local write "LED"(w99) -> ()
                          n233 = Multiply(x=w97, y=sgl 60.0) -> (x*y=w98:sgl)
                          n234 = Build Array(w89, w90, w91, w92, w93) -> (w88:sgl[])
                          n235 = Build Array "VS parameters"(w104, w108, w107, w106, w105, w98) -> (w124:dbl[])
                          n236 = local read "Pulse width (ms)"() -> (w128:sgl)
                          n237 = local read "Pulse delay (ms)"() -> (w127:sgl)
                          n238 = local read "Pulse period"() -> (w129:sgl)
                          n239 = local read "Pulse amp 0"() -> (w125:sgl)
                          n240 = local read "Pulse amp 1"() -> (w126:sgl)
                          n241 = local read "Pulse #"() -> (w130:sgl)
                          n242 = Build Array "LED parameters"(w100, w125, w126, w127, w128, w129, w130) -> (w123:sgl[])
                          n243 = Build Array (concatenate)(w124, w123, w88) -> (w114:dbl[])
                          n244 = Subtract(x=w114, y=w122) -> (x-y=w121:dbl[])
                          n245 = Absolute Value(x=w121) -> (abs(x)=w119:dbl[])
                          n246 = Less?(x=w119, y=1e-06) -> (x < y?=w118:bool[])
                          n247 = Array Size(array=w114) -> (size(s)=w110:i32)
                          n248 = for {
                            tunnel: w118 -> [w135] mode=indexing
                            shift-right: [w133] -> w117
                            shift-left: "" -> [w134]
                            tunnel: w114 -> [w132] mode=indexing
                            i -> [w131]
                            n249 = case shown="False" w135 {
                              tunnel: w134 -> [w143 w162]
                              tunnel: [w142 w162] -> w133
                              tunnel: w131 -> [w140 _]
                              tunnel: w132 -> [w136 _]
                              frame False {
                                n250 = case shown="17" w140 {
                                tunnel: ["dur" "ifi" "jit" "bkl" "fll" "tri" "led" "pai" "paf" "pdl" "pwd" "ppr" "pnm" "blk" "ori" "spf" "tpf" "ctr"] -> w139
                                frame 0, Default {
                                }
                                frame 1 {
                                }
                                frame 2 {
                                }
                                frame 3 {
                                }
                                frame 4 {
                                }
                                frame 5 {
                                }
                                frame 6 {
                                }
                                frame 7 {
                                }
                                frame 8 {
                                }
                                frame 9 {
                                }
                                frame 10 {
                                }
                                frame 11 {
                                }
                                frame 12 {
                                }
                                frame 13 {
                                }
                                frame 14 {
                                }
                                frame 15 {
                                }
                                frame 16 {
                                }
                                frame 17 {
                                }
                                }
                                n251 = Format Value(format string="%.3f", value (0)=w136) -> (output string=w137:string)  [unwired: 1 in]
                                n252 = call <vilib>:"Space Constant.vi"() -> ("String"=w141:string)
                                n253 = Concatenate Strings(w143, w139, w141, w137, w141) -> (w142:string)
                              }
                              frame True {
                              }
                            }
                          }
                          n254 = Reshape Array(w114, 1 ("dimension size"), w110) -> (w111:dbl[][])
                          n255 = Replace Array Subset(array=w113, new element=w111, index (row)=w94, index (col)=0) -> (w109:sgl[][])
                        }
                        frame #1 {
                          # "16"
                          n256 = local read "Manually give shock"() -> (w199:bool)
                          n257 = local read "Manually give water"() -> (w201:bool)
                          n258 = local read "Shock refractory period (ms)"() -> (w209:u32)
                          n259 = local read "Lick threshold (V)"() -> (w189:fxp<+,32,16>)
                          n260 = local read "Water refractory period (ms)"() -> (w211:u32)
                          n261 = local read "VS threshold (V)"() -> (w167:fxp<+,32,16>)
                          n262 = local read "Allow timeout"() -> (w203:bool)
                          n263 = local read "Give reward"() -> (w165:bool)
                          n264 = local read "Reward start delay (ms)"() -> (w213:u32)
                          n265 = local read "Allow shock"() -> (w205:bool)
                          n266 = local read "Save data"() -> (w197:bool)
                          n267 = local read "Shock duration (ms)"() -> (w210:u32)
                          n268 = local read "Track eye"() -> (w206:bool)
                          n269 = local read "Water duration (ms)"() -> (w212:u32)
                          n270 = local read "Reward period (ms)"() -> (w214:u32)
                          n271 = local read "Trial timeout (ms)"() -> (w208:u32)
                          n272 = Boolean To (0,1)(Boolean=w165) -> (0, 1=w164:i16)
                          n273 = Boolean To (0,1)(Boolean=w206) -> (0, 1=w207:i16)
                          n274 = Boolean To (0,1)(Boolean=w205) -> (0, 1=w204:i16)
                          n275 = Boolean To (0,1)(Boolean=w203) -> (0, 1=w202:i16)
                          n276 = Boolean To (0,1)(Boolean=w201) -> (0, 1=w200:i16)
                          n277 = Boolean To (0,1)(Boolean=w199) -> (0, 1=w198:i16)
                          n278 = Boolean To (0,1)(Boolean=w197) -> (0, 1=w196:i16)
                          n279 = To Single Precision Float(number=w189) -> (single precision float=w190:sgl)
                          n280 = To Single Precision Float(number=w167) -> (single precision float=w166:sgl)
                          n281 = Build Array "Beh parameters"(w214, w213, w212, w211, w210, w209, w208, w190, w207, w204, w202, w200, w198, w196, w166, w164) -> (w178:sgl[])
                          n282 = Subtract(x=w178, y=w195) -> (x-y=w194:dbl[])
                          n283 = Array Size(array=w178) -> (size(s)=w179:i32)
                          n284 = Absolute Value(x=w194) -> (abs(x)=w192:dbl[])
                          n285 = Less?(x=w192, y=1e-06) -> (x < y?=w191:bool[])
                          n286 = Reshape Array(w178, 1 ("dimension size"), w179) -> (w177:sgl[][])
                          n287 = local read "Total number of trials"() -> (w168:i32)
                          n288 = for {
                            tunnel: w191 -> [w231] mode=indexing
                            tunnel: w178 -> [w230] mode=indexing
                            shift-right: [w228] -> w187
                            shift-left: w188 -> [w229]
                            i -> [w232]
                            n289 = case shown="False" w231 {
                              tunnel: w232 -> [w240 _]
                              tunnel: w230 -> [w238 _]
                              tunnel: w229 -> [w235 w257]
                              tunnel: [w233 w257] -> w228
                              frame False {
                                n290 = case shown="15" w240 {
                                tunnel: ["rwp" "rwd" "wdr" "wre" "shd" "shr" "tto" "lkt" "etk" "ash" "ato" "gwt" "gsh" "sav" "vsh" "rew"] -> w234
                                frame 0, Default {
                                }
                                frame 1 {
                                }
                                frame 2 {
                                }
                                frame 3 {
                                }
                                frame 4 {
                                }
                                frame 5 {
                                }
                                frame 6 {
                                }
                                frame 7 {
                                }
                                frame 8 {
                                }
                                frame 9 {
                                }
                                frame 10 {
                                }
                                frame 11 {
                                }
                                frame 12 {
                                }
                                frame 13 {
                                }
                                frame 14 {
                                }
                                frame 15 {
                                }
                                }
                                n291 = Format Value(format string="%.3f", value (0)=w238) -> (output string=w236:string)  [unwired: 1 in]
                                n292 = call <vilib>:"Space Constant.vi"() -> ("String"=w237:string)
                                n293 = Concatenate Strings(w235, w234, w237, w236, w237) -> (w233:string)
                              }
                              frame True {
                              }
                            }
                          }
                          n294 = local read "Current trial #"() -> (w183:u16)
                          n295 = local read "run-stop"() -> (w175:bool)
                          n296 = local read "State Missed"() -> (w185:bool)
                          n297 = local read "VS missed"() -> (w184:bool)
                          n298 = Not(x=w175) -> (.not. x?=w174:bool)
                          n299 = Equal?(x=w183, y=w168) -> (x = y?=w186:bool)
                          n300 = Compound Arithmetic op=OR(w184, w185, w186) -> (w173:bool)
                          n301 = case shown="True" w173 {
                            frame False {
                            }
                            frame True {
                              w215 = FALSE
                              n302 = local write "Running!"(w215) -> ()
                              n303 = local write "run-stop"(w215) -> ()
                            }
                          }
                          n304 = Compound Arithmetic op=OR(w173, w174, w172) -> (w171:bool)
                          n305 = case shown="True" w171 {
                            tunnel: w187 -> [w222 _]
                            tunnel: [w218 w224] -> w170
                            tunnel: [FALSE TRUE] -> w163
                            frame False {
                              n306 = call <vilib>:"Space Constant.vi"() -> ("String"=w220:string)
                              n307 = Concatenate Strings(w222, "start", w220, "1.000", w220) -> (w218:string)
                              n308 = global write "Global 1.vi" "Start one trial"(TRUE) -> ()
                            }
                            frame True {
                              n309 = call <vilib>:"Space Constant.vi"() -> ("String"=w226:string)
                              n310 = Concatenate Strings("stop", w226, "1.000", w226) -> (w224:string)
                            }
                          }
                          n311 = Replace Array Subset(array=w181, new element=w177, index (row)=w169, index (col)=w182) -> (w176:sgl[][])
                        }
                        frame #2 {
                          n312 = case shown="False" w258 {
                            tunnel: w260 -> [w263 w264]
                            tunnel: [w262 w264] -> w259
                            frame False {
                              w261 = TRUE
                              n313 = Increment(x=w263) -> (x+1=w262:u16)
                              "Current trial #" <- w262
                              n314 = local write "VS busy"(w261) -> ()
                              n315 = local write "State busy"(w261) -> ()
                            }
                            frame True {
                            }
                          }
                        }
                      }
                      n316 = local read "Remote IP_Broadcast"() -> (w81:string)
                      n317 = local read "Remote port"() -> (w83:u16)
                      n318 = String To IP(1:w81) -> (0:w82:u32)
                      n319 = UDP Write(address=w82, port or service name=w83, connection ID=w79, data in=w70, 8:w80) -> (error out=w78:errorcluster, 3:w77:refnum<k16>)  [unwired: 1 in]
                    }
                    frame True {
                      n320 = stacked-sequence {
                        seq-local: [w285 _] -> [_ w381]
                        seq-local: [w284 _] -> [_ w382]
                        tunnel: w275 -> [w301 _]
                        tunnel: w274 -> [w292 _]
                        tunnel: w273 -> [w291 _]
                        tunnel: [_ w376] -> w272
                        tunnel: w271 -> [w290 _]
                        tunnel: [_ w373] -> w270
                        tunnel: [w278 _] -> w269
                        tunnel: [w286 _] -> w268
                        tunnel: w267 -> [_ w370]
                        tunnel: [_ w368] -> w266
                        frame #0 {
                          n321 = local read "Manually give shock"() -> (w311:bool)
                          n322 = local read "Manually give water"() -> (w313:bool)
                          n323 = local read "Shock refractory period (ms)"() -> (w321:u32)
                          n324 = local read "Lick threshold (V)"() -> (w302:fxp<+,32,16>)
                          n325 = local read "Water refractory period (ms)"() -> (w323:u32)
                          n326 = local read "VS threshold (V)"() -> (w282:fxp<+,32,16>)
                          n327 = local read "Allow timeout"() -> (w315:bool)
                          n328 = local read "Reward start delay (ms)"() -> (w325:u32)
                          n329 = local read "Allow shock"() -> (w317:bool)
                          n330 = local read "Save data"() -> (w309:bool)
                          n331 = local read "Shock duration (ms)"() -> (w322:u32)
                          n332 = local read "Track eye"() -> (w318:bool)
                          n333 = local read "Water duration (ms)"() -> (w324:u32)
                          n334 = local read "Reward period (ms)"() -> (w326:u32)
                          n335 = local read "Trial timeout (ms)"() -> (w320:u32)
                          n336 = Boolean To (0,1)(Boolean=w318) -> (0, 1=w319:i16)
                          n337 = Boolean To (0,1)(Boolean=w317) -> (0, 1=w316:i16)
                          n338 = Boolean To (0,1)(Boolean=w315) -> (0, 1=w314:i16)
                          n339 = Boolean To (0,1)(Boolean=w313) -> (0, 1=w312:i16)
                          n340 = Boolean To (0,1)(Boolean=w311) -> (0, 1=w310:i16)
                          n341 = Boolean To (0,1)(Boolean=w309) -> (0, 1=w308:i16)
                          n342 = To Single Precision Float(number=w302) -> (single precision float=w303:sgl)
                          n343 = To Single Precision Float(number=w282) -> (single precision float=w281:sgl)
                          n344 = local read "Give reward"() -> (w280:bool)
                          n345 = Boolean To (0,1)(Boolean=w280) -> (0, 1=w279:i16)
                          n346 = Build Array "Beh parameters"(w326, w325, w324, w323, w322, w321, w320, w303, w319, w316, w314, w312, w310, w308, w281, w279) -> (w286:sgl[])
                          n347 = Subtract(x=w286, y=w301) -> (x-y=w307:dbl[])
                          n348 = Absolute Value(x=w307) -> (abs(x)=w305:dbl[])
                          n349 = Less?(x=w305, y=1e-06) -> (x < y?=w304:bool[])
                          n350 = for {
                            tunnel: w304 -> [w341] mode=indexing
                            tunnel: w286 -> [w340] mode=indexing
                            shift-right: [w338] -> w287
                            shift-left: "" -> [w339]
                            i -> [w342]
                            n351 = case shown="False" w341 {
                              tunnel: w342 -> [w350 _]
                              tunnel: w340 -> [w348 _]
                              tunnel: w339 -> [w345 w367]
                              tunnel: [w343 w367] -> w338
                              frame False {
                                n352 = case shown="15" w350 {
                                tunnel: ["rwp" "rwd" "wdr" "wre" "shd" "shr" "tto" "lkt" "etk" "ash" "ato" "gwt" "gsh" "sav" "vst" "rew"] -> w344
                                frame 0, Default {
                                }
                                frame 1 {
                                }
                                frame 2 {
                                }
                                frame 3 {
                                }
                                frame 4 {
                                }
                                frame 5 {
                                }
                                frame 6 {
                                }
                                frame 7 {
                                }
                                frame 8 {
                                }
                                frame 9 {
                                }
                                frame 10 {
                                }
                                frame 11 {
                                }
                                frame 12 {
                                }
                                frame 13 {
                                }
                                frame 14 {
                                }
                                frame 15 {
                                }
                                }
                                n353 = Format Value(format string="%.3f", value (0)=w348) -> (output string=w346:string)  [unwired: 1 in]
                                n354 = call <vilib>:"Space Constant.vi"() -> ("String"=w347:string)
                                n355 = Concatenate Strings(w345, w344, w347, w346, w347) -> (w343:string)
                              }
                              frame True {
                              }
                            }
                          }
                          n356 = String Length(string=w287) -> (length=w288:i32)
                          n357 = Not Equal To 0?(x=w288) -> (x != 0?=w289:bool)
                          n358 = case shown="True" w289 {
                            tunnel: w291 -> [w327 w333]
                            tunnel: [w327 w332] -> w284
                            tunnel: w290 -> [w328 w331]
                            tunnel: [w328 w330] -> w285
                            tunnel: w287 -> [_ w329]
                            frame False {
                            }
                            frame True {
                              n359 = local read "Remote IP_Broadcast"() -> (w334:string)
                              n360 = local read "Remote port"() -> (w336:u16)
                              n361 = String To IP(1:w334) -> (0:w335:u32)
                              n362 = UDP Write(address=w335, port or service name=w336, connection ID=w331, data in=w329, 8:w333) -> (error out=w332:errorcluster, 3:w330:refnum<k16>)  [unwired: 1 in]
                            }
                          }
                          n363 = local read "Total number of trials"() -> (w283:i32)
                          n364 = local read "Current trial #"() -> (w296:u16)
                          n365 = local read "run-stop"() -> (w295:bool)
                          n366 = local read "State Missed"() -> (w298:bool)
                          n367 = local read "VS missed"() -> (w297:bool)
                          n368 = Not(x=w295) -> (.not. x?=w294:bool)
                          n369 = Equal?(x=w296, y=w283) -> (x = y?=w299:bool)
                          n370 = Compound Arithmetic op=OR(w297, w298, w299) -> (w293:bool)
                          n371 = Compound Arithmetic op=OR(w293, w294, w292) -> (w278:bool)
                          n372 = case shown="True" w278 {
                            frame False {
                            }
                            frame True {
                              w337 = FALSE
                              n373 = local write "Running!"(w337) -> ()
                              n374 = local write "run-stop"(w337) -> ()
                            }
                          }
                        }
                        frame #1 {
                          n375 = UDP Read(connection ID=w381, timeout ms (25000)=0, 8:w382) -> (data out=w369:string, error out=w377:errorcluster, 3:w373:refnum<k16>, 6:w371:u32)  [unwired: 1 in, 1 out]
                          n376 = Unbundle By Name(w377) -> ("code"=w378:i32)
                          n377 = Equal?(x=w378, y=56) -> (x = y?=w380:bool)
                          n378 = case shown="True" w380 {
                            tunnel: w377 -> [w422 _]
                            tunnel: [w422 errorcluster {"status"=FALSE, "code"=0, "source"=""} ("error out")] -> w376
                            frame False {
                            }
                            frame True {
                            }
                          }
                          n379 = String Length(string=w369) -> (length=w375:i32)
                          n380 = Not Equal To 0?(x=w375) -> (x != 0?=w374:bool)
                          n381 = case shown="True" w374 {
                            tunnel: w371 -> [_ w387]
                            tunnel: w370 -> [w383 w386]
                            tunnel: w369 -> [_ w391]
                            tunnel: [w383 w384] -> w368
                            frame False {
                            }
                            frame True {
                              (unwired) -1.0 ("default value 2")
                              (unwired) "no" ("default value 1")
                              n382 = Scan From String(format string="%s %f ", input string=w391, initial scan location=u32 0) -> (output 1=w388:string, output 2=w385:dbl)  [unwired: 3 in, 3 out]
                              n383 = case shown="\"TrlDone\", Default" w388 {
                                tunnel: w387 -> [w399]
                                tunnel: w386 -> [w392]
                                tunnel: w385 -> [w394]
                                tunnel: [w392] -> w384
                                frame "TrlDone", Default {
                                n384 = local read "Remote IP_State machine"() -> (w396:string)
                                n385 = IP To String(1:TRUE ("dot notation? (F)"), 2:w399) -> (0:w393:string)
                                "Originating IP" <- w393
                                n386 = Match True/False String(2:"" ("false string"), 3:w396, 4:w393) -> (0:w395:bool)  [unwired: 1 out]
                                n387 = case shown="False" w395 {
                                tunnel: w392 -> [w400 w419]
                                tunnel: w394 -> [w401 w420]
                                tunnel: w393 -> [w405 _]
                                frame False {
                                n388 = local read "Remote IP_Visual stimulation"() -> (w403:string)
                                n389 = Match True/False String(2:"" ("false string"), 3:w403, 4:w405) -> (0:w402:bool)  [unwired: 1 out]
                                n390 = case shown="True" w402 {
                                tunnel: w401 -> [_ w410]
                                tunnel: w400 -> [_ w409]
                                frame False {
                                "Error 2" <- "Unknown source Error"
                                }
                                frame True {
                                n391 = Subtract(x=w410, y=w409) -> (x-y=w413:dbl)
                                n392 = global write "Global 1.vi" "camera stop"(TRUE ("dot notation? (F)")) -> ()
                                n393 = Absolute Value(x=w413) -> (abs(x)=w412:dbl)
                                n394 = local write "VS busy"(FALSE) -> ()
                                n395 = Greater?(x=w412, y=1e-06) -> (0:→"VS missed":bool)
                                }
                                }
                                }
                                frame True {
                                n396 = Subtract(x=w420, y=w419) -> (x-y=w418:dbl)
                                n397 = local write "State busy"(FALSE) -> ()
                                n398 = Absolute Value(x=w418) -> (abs(x)=w417:dbl)
                                n399 = Greater?(x=w417, y=1e-06) -> (0:→"State Missed":bool)
                                }
                                }
                                }
                              }
                              "Incoming data" <- w391
                            }
                          }
                        }
                      }
                    }
                  }
                  n400 = node-c288() -> ()  [unwired: 1 in, 1 out]
                }
                n401 = node-c288(w39) -> ()  [unwired: 1 out]
                n402 = To Single Precision Float(number=w29) -> (single precision float=w24:sgl[][])
                n403 = local read "Save data"() -> (w27:bool)
                n404 = UDP Close(connection ID=w18, 8:w17) -> (error out=w22:errorcluster)  [unwired: 1 out]
                n405 = case shown="True" w27 {
                  tunnel: w26 -> [w428 w444]
                  tunnel: w25 -> [_ w443]
                  tunnel: w24 -> [_ w435]
                  tunnel: [w428 w432] -> w21
                  tunnel: w16 -> [_ w431]
                  frame False {
                  }
                  frame True {
                    n406 = Add(x=w431, y=2) -> (x+y=w429:i32)
                    n407 = Multiply(x=w429, y=4) -> (x*y=w440:i32)
                    n408 = Set File Position(offset (in bytes) (0)=w440, refnum=w443, from (0:start)=enum16{"start", "end", "current"}."start", error in=w444) -> (refnum out=w437:refnum<file>, error out=w438:errorcluster)
                    n409 = Write to Binary File(file (use dialog)=w437, data=w435, error in=w438, 5:FALSE ("prepend array or string size? (T)"), 9:T5."little-endian" ("byte order (0:big-endian, network order)")) -> (refnum out=w433:refnum<file>, error out=w434:errorcluster)  [unwired: 1 in, 1 out]
                    n410 = Close File(refnum=w433, error in=w434) -> (error out=w432:errorcluster)  [unwired: 1 out]
                  }
                }
                n411 = Merge Errors(w22, w21) -> (w20:errorcluster)
                n412 = stacked-sequence {
                  tunnel: w20 -> [w41]
                  frame #0 {
                    n413 = call <vilib>:"Simple Error Handler.vi"("error in (no error)"=w41) -> ()  [unwired: 4 in, 5 out]
                  }
                }
              }
              frame 2 {
              }
            }
          }
          frame #2 {
            n414 = Wait (ms)(milliseconds to wait=u32 100) -> ()  [unwired: 1 out]
          }
        }
      }
    }
  }
